vi "Evaluate Severity.vi"(10 "error in (no error)":errorcluster) -> (2 "Severity":T1)   [LabVIEW 2018]
doc: "Evaluates the severity of the error"
uses:
  Error Severity.ctl
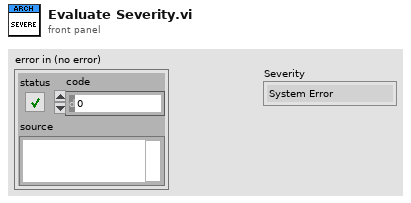
[diagram p1: front panel]
types:
  T1 = typedef "Error Severity.ctl" = enum16{"System Error", "Wash Error", "Minor"}
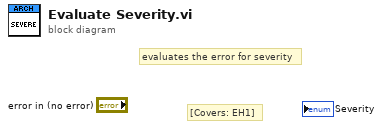
[diagram p0: block diagram]
diagram:
  # "[Covers: EH1]"
  # "evaluates the error for severity"
